vi "Stop Core.vi"(10 "final error code":i32, 11 "AIO in":refnum<class "AIO.lvclass">) -> (3 "AIO out":refnum<class "AIO.lvclass">)   [LabVIEW 2024, in "AIO Actor.lvlib" / "AIO.lvclass"]
doc: "(<B>Filename</B>: Actor Framework.lvlib:Actor.lvclass:Stop Core.vi)\n\nDefines what the actor does before it stops. Use the <B>final error code</B> input to determine whether the actor shut down in response to an error.\n\nBy default, this method does nothing. A descendant class may override it to define behavior, such as shutting down any processes the actor initiated in its override of the Actor Core method."
uses:
  AIO.lvclass
  AIO.lvclass/AIO.ctl
  <vilib>/ActorFramework/Actor/Actor.lvclass
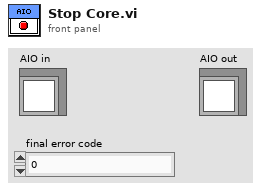
[diagram p1: front panel]
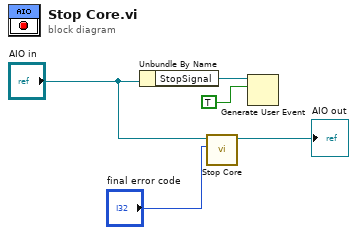
[diagram p0: block diagram]
diagram:
  n1 = Unbundle By Name("AIO in") -> ("StopSignal"=w2:refnum<user-event>)
  n2 = call-parent "Stop Core.vi"("final error code"="final error code", "Actor in"="AIO in") -> ("Actor out"=→"AIO out":refnum<class "AIO.lvclass">)  [unwired: 9 in]
  n3 = Generate User Event(user event=w2, event data cluster=TRUE ("event data")) -> ()  [unwired: 2 in, 2 out]
